vi "unitech.vi"() -> ()   [LabVIEW 2014]
panel:
  out "Response":string="C489TV_BG-206365_WT20060278"
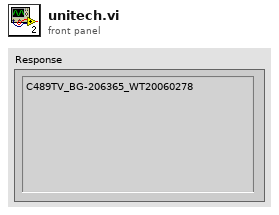
[diagram p1: front panel]
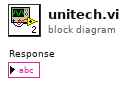
[diagram p0: block diagram]
diagram:
